vi "tcpIP.vi"() -> ()   [LabVIEW 2023]
uses:
  <extravilib>/ChannelInstances/Stream-str.lvlib
panel:
  in  "stop":bool
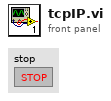
[diagram p1: front panel]
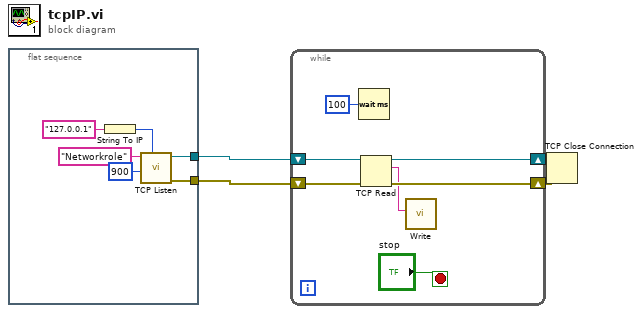
[diagram p0: block diagram]
diagram:
  n1 = flat-sequence {
    tunnel: [w10] -> w2
    tunnel: [w9] -> w1
    frame #0 {
      n2 = String To IP(1:"127.0.0.1" ("name")) -> (0:w8:u32)
      n3 = call <vilib>:"TCP Listen.vi"("net address"=w8, "port"=u16 900, "service name"="Networkrole") -> ("error out"=w9:errorcluster, "connection ID"=w10:refnum<k5>)  [unwired: 4 in, 3 out]
    }
  }
  n4 = while {
    shift-right: [w17] -> w4
    shift-left: w2 -> [w15]
    shift-right: [w16] -> w3
    shift-left: w1 -> [w14]
    stop <- "stop" stop-if-true
    n5 = Wait (ms)(milliseconds to wait=u32 100) -> ()  [unwired: 1 out]
    n6 = TCP Read(connection ID=w15, error in (no error)=w14) -> (connection ID out=w17:refnum<k5>, data out=w11:string, error out=w16:errorcluster)  [unwired: 3 in]
    n7 = call <extravilib>:"Write.vi"("element"=w11) -> ()  [unwired: 8 in, 3 out]
  }
  n8 = TCP Close Connection(connection ID=w4, error in (no error)=w3) -> ()  [unwired: 1 in, 2 out]
